vi "位置范围设定VI.vi"(10 "x":dbl, 11 "位置1":cluster{"上限":dbl, "下限":dbl}={"上限"=726.0, "下限"=686.0}) -> (3 "1":bool)   [LabVIEW 2017]
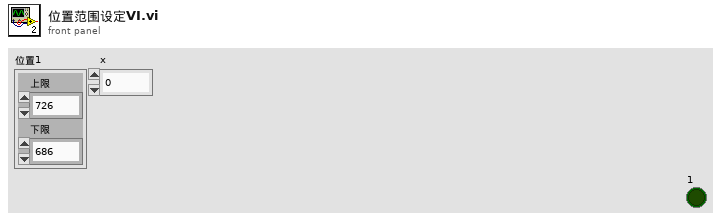
[diagram p1: front panel]
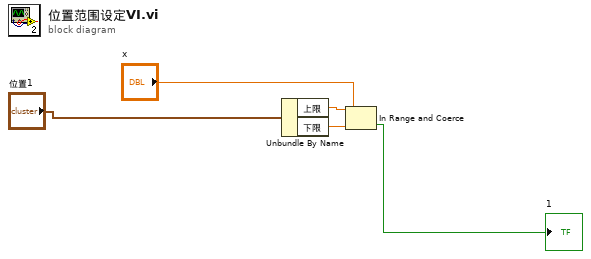
[diagram p0: block diagram]
diagram:
  n1 = Unbundle By Name("位置1") -> ("上限"=w5:dbl, "下限"=w4:dbl)
  n2 = In Range and Coerce(upper limit=w5, x="x", lower limit=w4) -> (In Range?=→"1":bool)  [unwired: 1 out]
